vi "MainGui-ProductListUpdate.vi"(8 "error in (no error)":errorcluster) -> (0 "error out":errorcluster)   [LabVIEW 2016]
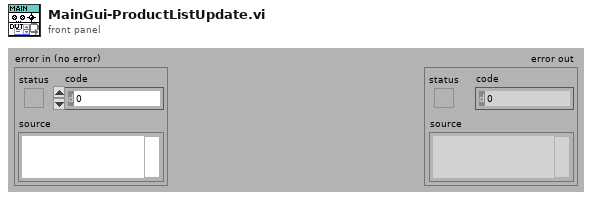
[diagram p1: front panel]
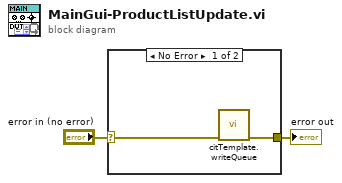
[diagram p0: block diagram]
diagram:
  n1 = case shown="No Error" "error in (no error)" {
    selector: "error in (no error)" -> [w3 w5]
    tunnel: [w4 w5] -> w1
    frame No Error {
      n2 = call "citTemplate.writeQueue.vi"("error in (no error)"=w3) -> ("error out"=w4:errorcluster)  [unwired: 14 in]
    }
    frame Error {
    }
  }
  "error out" <- w1
